vi "U3 Single Pulse Bit Output (no-timer).vi"() -> ()   [LabVIEW 2021]
panel:
  in  "Digital I/O Channel":i32=4
  in  "Pulse Type":bool=TRUE
  in  "Pulse Time (microseconds)":i32=100000
  out "Error Message":string
  out "error out":errorcluster
  # "Uses the PUT_WAIT IOType to create a single pulse on a digital output line on the U3.\n\nThe put_wait works by adding a delay between two events within a low-level Feedback\ncommand.  In the UD driver, if you add a request to set FIO0 high, add a request to wait\n100000 microseconds, add a request to set FIO0 low, and then Go, these will be sent in\na single low-level Feedback command, creating a 100 ms positive pulse on FIO0."
  # "0-7       FIO0-FIO7\n8-15     EIO0-EIO7\n16-19   CIO0-CIO3"
  # "Range is 0-8388480.\nActual resolution is 128 us.\nActual minimum is about 30 us."
  # "High Pulse\n\nLow Pulse"
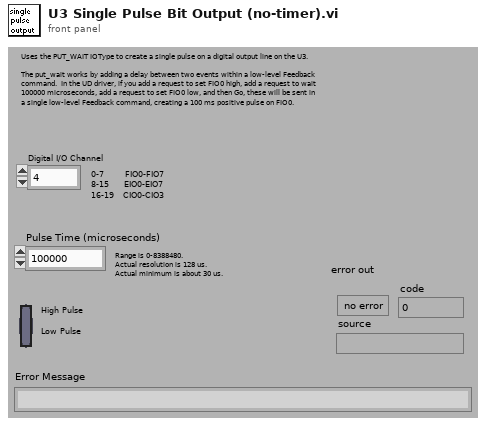
[diagram p1: front panel]
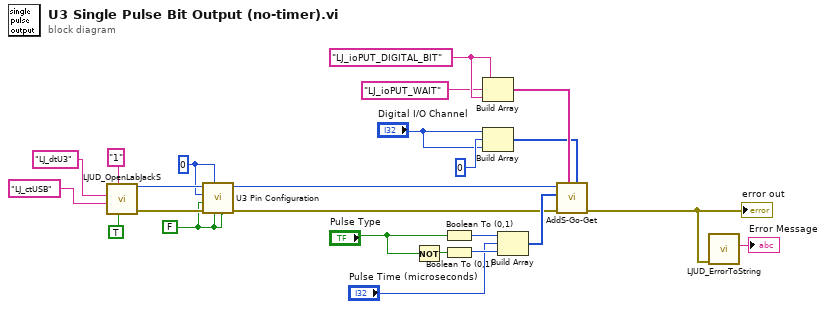
[diagram p0: block diagram]
diagram:
  w13 = FALSE ("Enable Counter0")
  w1 = 0 ("FIO/EIO Analog Enable")
  w12 = "LJ_ioPUT_DIGITAL_BIT" ("IOType")
  n1 = call "LJUD_OpenLabJackS.vi"("FirstFound"=TRUE, "Address"="1", "ConnectionType"="LJ_ctUSB", "DeviceType"="LJ_dtU3") -> ("error out"=w16:errorcluster, "Handle"=w17:i32)  [unwired: 5 in, 1 out]
  n2 = call "U3 Pin Configuration.vi"("Enable Counter1"=w13, "Enable Counter0"=w13, "FIO/EIO Analog Enable"=w1, "error in"=w16, "Enable DAC1"=w13, "Number of Timers Enabled"=w1, "Handle In"=w17) -> ("error out"=w15:errorcluster, "Handle Out"=w14:i32)  [unwired: 3 in]
  n3 = Not(x="Pulse Type") -> (.not. x?=w6:bool)
  n4 = Boolean To (0,1)(Boolean="Pulse Type") -> (0, 1=w4:i16)
  n5 = Boolean To (0,1)(Boolean=w6) -> (0, 1=w3:i16)
  n6 = Build Array(w12, "LJ_ioPUT_WAIT" ("Input Element"), w12) -> (w10:string[])
  n7 = Build Array("Digital I/O Channel", 0, "Digital I/O Channel") -> (w8:i32[])
  n8 = Build Array(w4, "Pulse Time (microseconds)", w3) -> (w22:i32[])
  n9 = call "AddS-Go-Get.vi"("Channels"=w8, "IOTypes"=w10, "error in"=w15, "Values Write"=w22, "Handle In"=w14) -> ("error out"=w23:errorcluster)  [unwired: 4 in, 2 out]
  "error out" <- w23
  n10 = call "LJUD_ErrorToString.vi"("error in"=w23) -> ("String"=→"Error Message":string)  [unwired: 10 in]
